vi "Noise Exposure.vi"() -> ()   [LabVIEW 2021]
uses:
  <vilib>/Platform/TimedLoop/XDataNode/wakeup.ctl
  <vilib>/Platform/TimedLoop/XDataNode/XDNodeRunTimeDep.lvlib
  <vilib>/Platform/TimedLoop/XDataNode/nitl_modes.ctl
  <vilib>/Platform/TimedLoop/XDataNode/timing_clust.ctl
  <vilib>/Platform/TimedLoop/XDataNode/XDataNode.xnode
  <vilib>/myRIO/Instrument Drivers/Utilities/Utilities.lvlib
panel:
  in  "Stop Button":bool
  in  "Tab Control":enum32{"Noise Exposure", "Custom Graphs"}(tab)
  in  "Graph Time Max":dbl=5.0
  in  "Graph Time Min":dbl
  out "Microphone":waveform(dbl)(graph)
  in  "Seconds to Record":dbl=2.0 min=0.0 step=0.1
  out "Request Exceeds \n100,000 samples":bool
  in  "Collect Data":bool
  out "Acquiring":bool
  out "Pk-Pk":dbl format="%.2p"
  out "RMS":dbl format="%.2p"
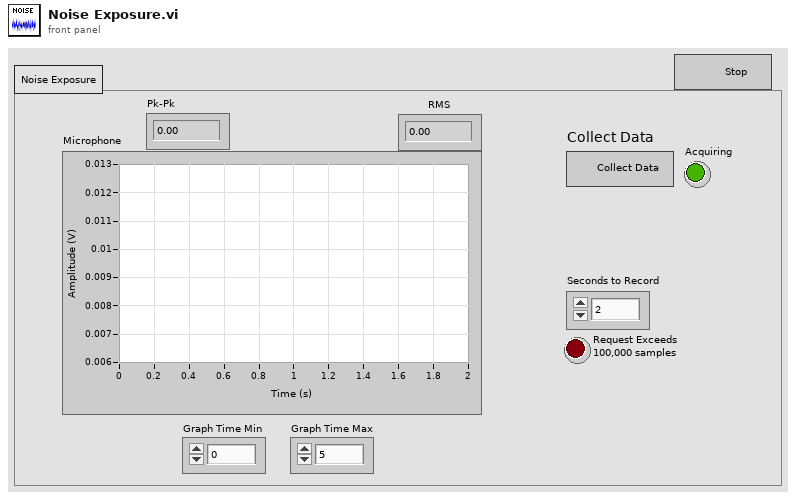
[diagram p1: front panel]
types:
  T1 = typedef "XDNodeRunTimeDep.lvlib/timing_clust.ctl" = cluster{"Expected End [f-1]":u64, "Actual End [f-1]":u64, "Finished Late? [f-1]":bool, "Expected End [i-1]":u64, "Actual End [i-1]":u64, "Finished Late? [i-1]":bool, "Expected Start [i]":u64, "Actual Start [i]":u64, "Expected Start [f]":u64, "Actual Start [f]":u64, "Source Name":string, "Structure Name":string, "Period":i64, "Deadline":i64, "Offset":i64, "Start":i64, "Priority":i32, "Timeout":i32, "Mode":T2, "Wakeup Reason":T3, "Error":errorcluster, "Source Type":string, "Secondary Source Type":string, "Global End Time":u64, "Global Start Time":u64, "Frame Duration":u64, "Iteration Duration":u64, "Assigned CPU":i32, "I/O Scan Engine Mode":u32}
  T2 = typedef "XDNodeRunTimeDep.lvlib/nitl_modes.ctl" = enum32{"No Change", "Process missed periods, maintain original phase", "Discard missed periods, maintain original phase", "Process missed periods, ignore original phase", "Discard missed periods, ignore original phase"}
  T3 = typedef "XDNodeRunTimeDep.lvlib/wakeup.ctl" = enum32{"Normal", "Aborted", "Asynchronous wakeup", "Timing source error", "Timed loop error", "Timeout"}
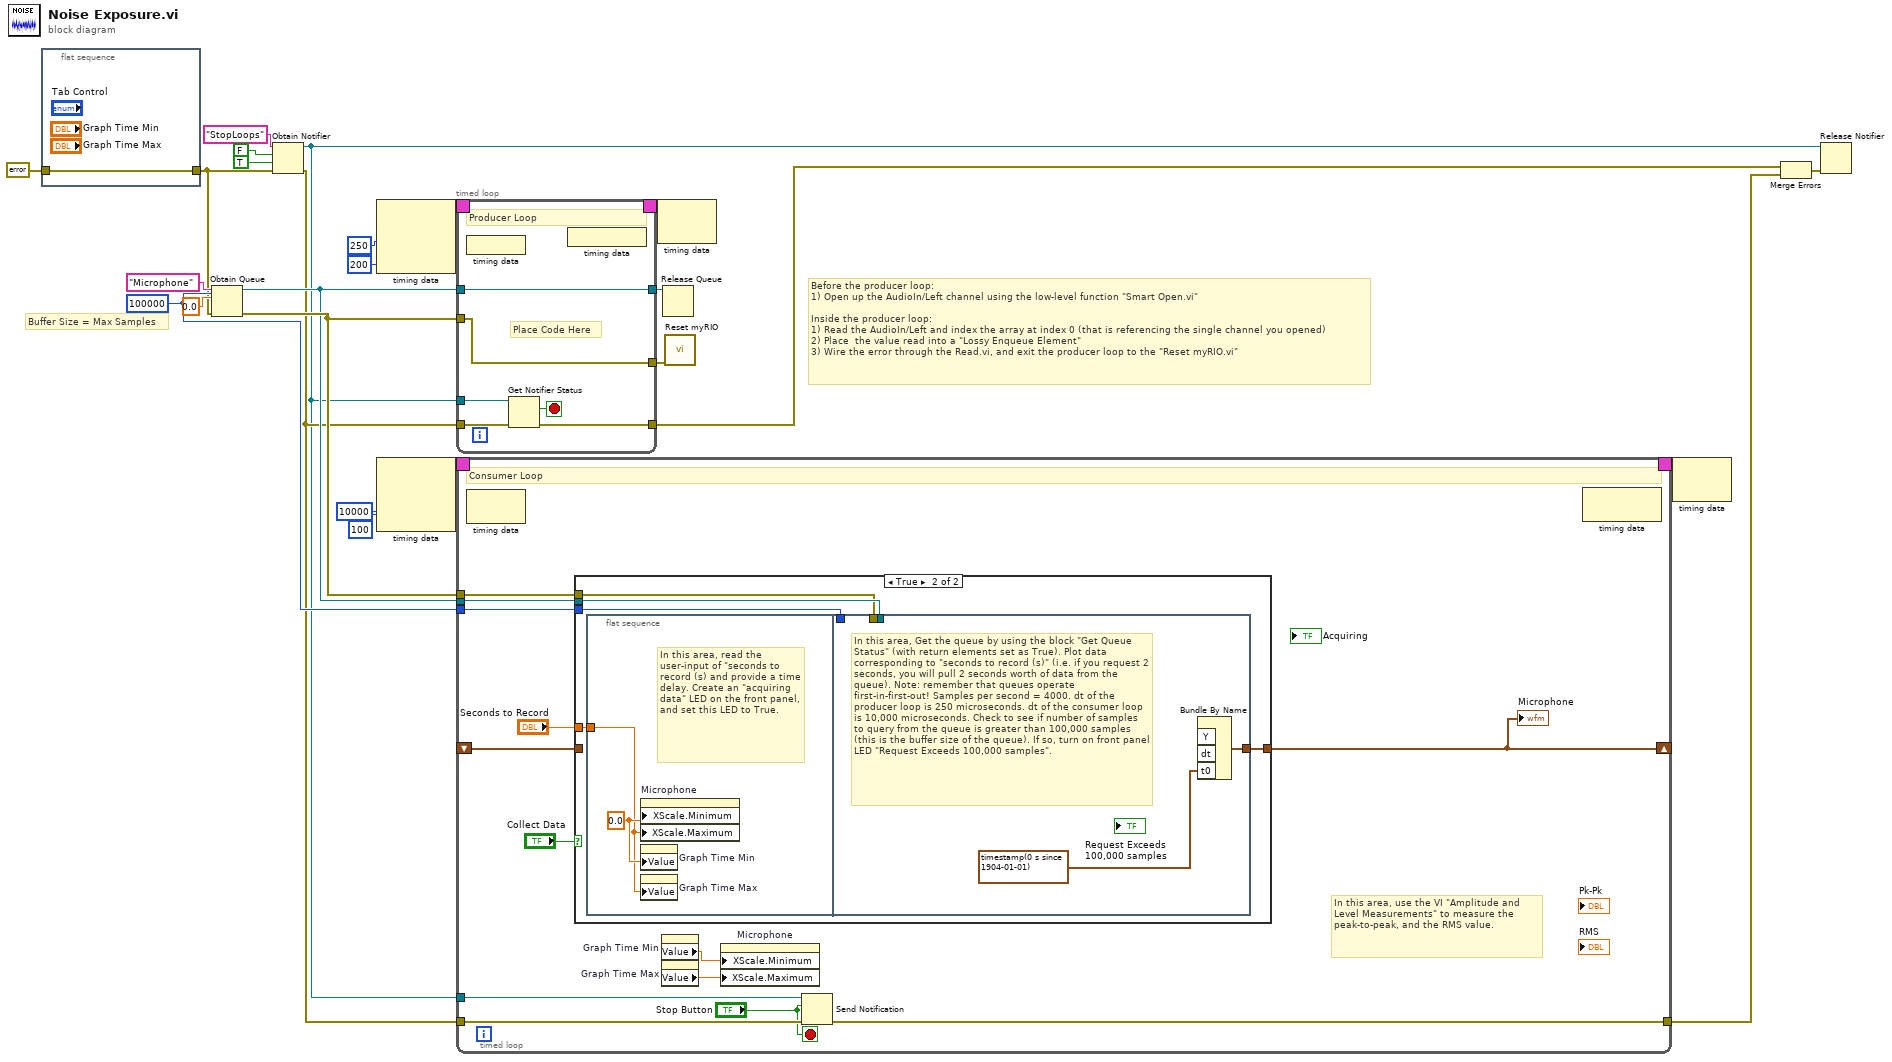
[diagram p0: block diagram]
diagram:
  w7 = 100000 ("max queue size (-1, unlimited)")
  # "Before the producer loop:\n1) Open up the AudioIn/Left channel using the low-level function \"Smart Open.vi\"\n\nInside the producer loop:\n1) Read the AudioIn/Left and index the array at index 0 (that is referencing the single channel you opened)\n2) Place  the value read into a \"Lossy Enqueue Element\"\n3) Wire the error through the Read.vi, and exit the producer loop to the \"Reset myRIO.vi\""
  # "Buffer Size = Max Samples"
  n1 = flat-sequence {
    tunnel: errorcluster {"status"=FALSE, "code"=0, "source"=""} ("error in") -> [w26]
    tunnel: [w26] -> w5
    frame #0 {
    }
  }
  n2 = Obtain Queue(max queue size (-1, unlimited)=w7, name (unnamed)="Microphone", element data type=0.0 ("x-y"), error in (no error)=w5) -> (queue out=w3:refnum<queue>, error out=w4:errorcluster)  [unwired: 1 in, 1 out]
  n3 = Obtain Notifier(name (unnamed)="StopLoops", notification data type=FALSE ("Stop Button"), create if not found? (T)=TRUE, error in (no error)=w5) -> (notifier out=w1:refnum<notifier>, error out=w2:errorcluster)  [unwired: 1 out]
  n4 = node-c288(i64 250 ("Period"), 200 ("Priority")) -> (w25:T1)  [unwired: 1 in]
  n5 = node-c288(i64 10000 ("Period"), 100 ("Priority")) -> (w14:T1)  [unwired: 1 in]
  n6 = timed-loop "Timed Loop" {
    timing: w25 -> [_]
    timing-out: [_] -> w24
    tunnel: w4 -> [w27]
    tunnel: [w27] -> w16
    tunnel: w3 -> [w28]
    tunnel: [w28] -> w21
    tunnel: w2 -> [w31]
    tunnel: [w30] -> w11
    tunnel: w1 -> [w32]
    stop <- w29 stop-if-true
    # "Place Code Here"
    # "Producer Loop"
    n7 = node-c288() -> ()  [unwired: 1 in]
    n8 = Get Notifier Status(notifier=w32, error in (no error)=w31) -> (current notification=w29:bool, error out=w30:errorcluster)  [unwired: 3 out]
    n9 = node-c288() -> ()  [unwired: 1 out]
  }
  n10 = timed-loop {
    tunnel: w2 -> [w40]
    tunnel: w1 -> [w41]
    tunnel: [w39] -> w10
    tunnel: w7 -> [w45]
    tunnel: w3 -> [w46]
    shift-right: [w36] -> _
    shift-left: _ -> [w47]
    timing: w14 -> [_]
    timing-out: [_] -> w13
    tunnel: w4 -> [w37]
    stop <- "Stop Button" stop-if-true
    # "In this area, use the VI \"Amplitude and Level Measurements\" to measure the peak-to-peak, and the RMS value."
    # "Consumer Loop"
    n11 = node-c288() -> ()  [unwired: 1 in, 1 out]
    n12 = case shown="True" "Collect Data" {
      tunnel: [w50 w55] -> w36
      tunnel: w47 -> [w50 _]
      tunnel: w46 -> [_ w54]
      tunnel: w45 -> [_ w53]
      tunnel: w37 -> [_ w52]
      tunnel: "Seconds to Record" -> [_ w51]
      frame False {
      }
      frame True {
        n13 = flat-sequence {
          tunnel: w51 -> [w56]
          tunnel: w53 -> [_]
          tunnel: w54 -> [_]
          tunnel: [w59] -> w55
          tunnel: w52 -> [_]
          frame #0 {
            w57 = 0.0 ("X Scale.Range:Minimum")
            # "In this area, read the user-input of \"seconds to record (s) and provide a time delay. Create an \"acquiring data\" LED on the front panel, and set this LED to True."
            n14 = property on="Microphone" class="WFGraph (strict)"("XScale.Minimum"=w57, "XScale.Maximum"=w56) -> ()  [unwired: 2 in, 2 out]
            n15 = property on="Graph Time Min" class="DigNum (strict)"("Value"=w57) -> ()  [unwired: 2 in, 2 out]
            n16 = property on="Graph Time Max" class="DigNum (strict)"("Value"=w56) -> ()  [unwired: 2 in, 2 out]
          }
          frame #1 {
            # "In this area, Get the queue by using the block \"Get Queue Status\" (with return elements set as True). Plot data corresponding to \"seconds to record (s)\" (i.e. if you request 2 seconds, you will pull 2 seconds worth of data from the queue). Note: remember that queues operate first-in-first-out! Samples per second = 4000. dt of the producer loop is 250 microseconds. dt of the consumer loop is 10,000 microseconds. Check to see if number of samples to query from the queue is greater than 100,000 samples (this is the buffer size of the queue). If so, turn on front panel LED \"Request Exceeds 100,000 samples\"."
            n17 = Bundle By Name("t0"=timestamp(0 s since 1904-01-01)) -> (w59:waveform(dbl))  [unwired: 3 in]
          }
        }
      }
    }
    "Microphone" <- w36
    n18 = property on="Graph Time Min" class="DigNum (strict)"() -> ("Value"=w42:dbl)  [unwired: 2 in, 2 out]
    n19 = property on="Graph Time Max" class="DigNum (strict)"() -> ("Value"=w43:dbl)  [unwired: 2 in, 2 out]
    n20 = property on="Microphone" class="WFGraph (strict)"("XScale.Minimum"=w42, "XScale.Maximum"=w43) -> ()  [unwired: 2 in, 2 out]
    n21 = Send Notification(notification="Stop Button", notifier=w41, error in (no error)=w40) -> (error out=w39:errorcluster)  [unwired: 1 out]
    n22 = node-c288() -> ()  [unwired: 1 in, 1 out]
  }
  n23 = node-c288(w24) -> ()  [unwired: 1 out]
  n24 = Release Queue(queue=w21) -> ()  [unwired: 2 in, 3 out]
  n25 = call <vilib>:"Reset myRIO.vi"("error in (no error)"=w16) -> ()  [unwired: 10 in, 1 out]
  n26 = node-c288(w13) -> ()  [unwired: 1 out]
  n27 = Merge Errors(w11, w10) -> (w17:errorcluster)
  n28 = Release Notifier(notifier=w1, error in (no error)=w17) -> ()  [unwired: 1 in, 3 out]
